vi "data acquistion.vi"() -> ()   [LabVIEW 2018]
panel:
  out "current time 2":timestamp
  out "current time":timestamp
  out "Numeric Indicator":dbl
  in  "Numeric Control":dbl
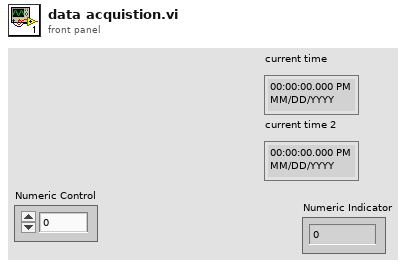
[diagram p1: front panel]
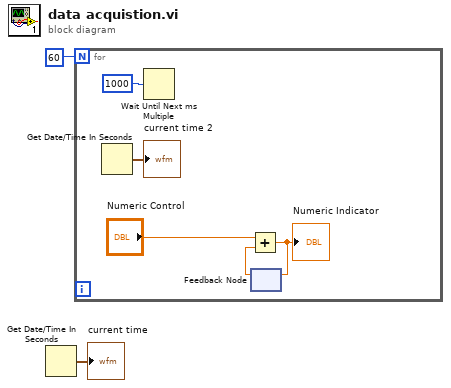
[diagram p0: block diagram]
diagram:
  n1 = Get Date/Time In Seconds() -> (seconds since 1Jan1904=→"current time":timestamp)
  n2 = for {
    N: 60 -> [_]
    n3 = Get Date/Time In Seconds() -> (seconds since 1Jan1904=→"current time 2":timestamp)
    n4 = Wait Until Next ms Multiple(millisecond multiple=u32 1000) -> ()  [unwired: 1 out]
    n5 = feedback #1() -> (w6:dbl)  [unwired: 1 in]
    n6 = Add(x="Numeric Control", y=w6) -> (x+y=w4:dbl)
    "Numeric Indicator" <- w4
    n7 = feedback-in #1(w4) -> ()
  }
